vi "Read Passwords.vi"(1 "Path to Password files...":path) -> (0 "Result":string)   [LabVIEW 2020]
panel:
  # "This VI looks for files that end in \"password.txt\" and adds the rightmost\nwords to LabVIEW's password cache.\nIf you want to specify more passwords, you can add them in \n\"my passwords.txt\" or \"more passwords.txt\"."
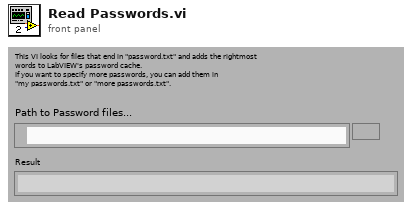
[diagram p1: front panel]
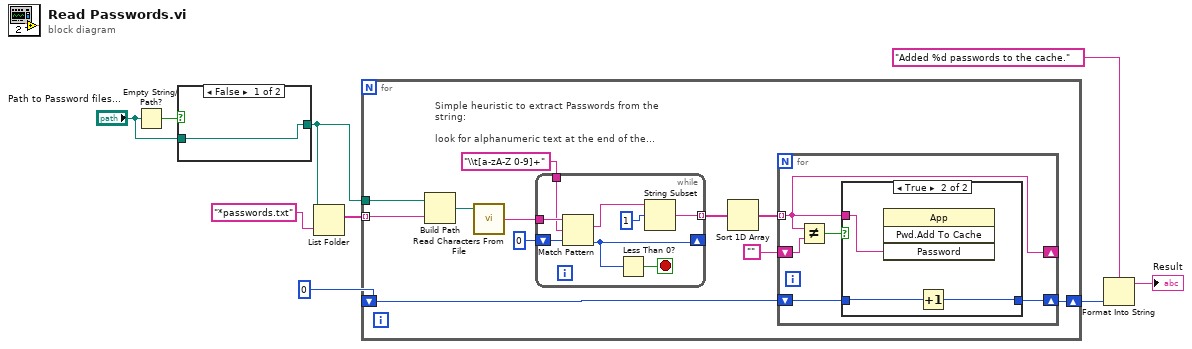
[diagram p0: block diagram]
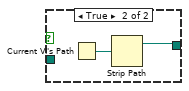
[diagram p2: hidden frame]
diagram:
  n1 = Empty String/Path?(string/path="Path to Password files...") -> (empty?=w2:bool)
  n2 = case shown="False" w2 {
    tunnel: [w10 w12] -> w3
    tunnel: "Path to Password files..." -> [w10 _]
    frame False {
    }
    frame True {
      n3 = Current VI's Path() -> (path=w11:path)
      n4 = Strip Path(path=w11) -> (stripped path=w12:path)  [unwired: 1 out]
    }
  }
  n5 = List Folder(path=w3, pattern="*passwords.txt") -> (filenames=w8:string[])  [unwired: 2 in, 3 out]
  n6 = for {
    tunnel: w8 -> [w22] mode=indexing
    tunnel: w3 -> [w23]
    shift-right: [w13] -> w4
    shift-left: 0 -> [w14]
    n7 = Build Path(base path=w23, name or relative path=w22) -> (appended path=w21:path)
    n8 = call <vilib>:"Read Characters From File.vi"("file path (dialog if empty)"=w21) -> ("character string"=w18:string)  [unwired: 5 in, 3 out]
    n9 = while "Simple heuristic to extract Passwords from the string:\n\nlook for alphanumeric text at the end of the line that is\npreceded by a tab character." {
      tunnel: w18 -> [w40]
      shift-right: [w37] -> _
      shift-left: 0 -> [w39]
      tunnel: [w34] -> w17 mode=indexing
      tunnel: "\\t[a-zA-Z 0-9]+" -> [w33]
      stop <- w38 stop-if-true
      n10 = Match Pattern(string=w40, regular expression=w33, offset (0)=w39) -> (match substring=w36:string, offset past match=w37:i32)  [unwired: 2 out]
      n11 = Less Than 0?(x=w37) -> (x < 0?=w38:bool)
      n12 = String Subset(string=w36, offset (0)=1) -> (substring=w34:string)  [unwired: 1 in]
    }
    n13 = Sort 1D Array(array=w17) -> (sorted array=w16:string[])
    n14 = for {
      tunnel: w16 -> [w26] mode=indexing
      shift-right: [w26] -> _
      shift-left: "" -> [w28]
      shift-right: [w25] -> w13
      shift-left: w14 -> [w24]
      n15 = Not Equal?(x=w26, y=w28) -> (x != y?=w27:bool)
      n16 = case shown="True" w27 {
        tunnel: w26 -> [_ w32]
        tunnel: [w29 w30] -> w25
        tunnel: w24 -> [w29 w31]
        frame False {
        }
        frame True {
          n17 = invoke class="App" method="Pwd.Add To Cache"("Password"=w32) -> ()  [unwired: 3 in, 4 out]
          n18 = Increment(x=w31) -> (x+1=w30:i32)
        }
      }
    }
  }
  n19 = Format Into String(format string="Added %d passwords to the cache.", w4) -> (resulting string=→"Result":string)  [unwired: 2 in, 1 out]
